vi "Teleop.vi"(10 "Match Info":T1={"Autonomous Elapsed Seconds"=0.0, "TeleOp Elapsed Seconds"=0.0, "Disabled Elapsed Seconds"=0.0, "Visited Autonomous"=FALSE, "Visited TeleOp"=FALSE, "Visited Disabled"=FALSE, "Autonomous Settings"={"Autonomous Style"=enum."Independent", "VI Refnum"=refnum}}, 11 "Call Context":T2) -> ()   [LabVIEW 2013]
doc: "This VI is called for each TeleOp packet received from the DS where the robot is not disabled. It is often used to read from the joysticks and update I/O or to update setpoints for timed control loops. It should complete and return within 20 milliseconds or it may miss DS packets."
uses:
  <vilib>/Rock Robotics/WPI/DriverStation/WPI_DriverStationDerivedRobotMode.ctl
  <vilib>/Rock Robotics/WPI/DriverStation/WPI_DriverStationMatch Info.ctl
  RefnameEnum.ctl
  LEDSaction.ctl
  Robot Global Data.vi
  <vilib>/Rock Robotics/WPI/Joystick/WPI_JoystickGetSetRefNum.vi
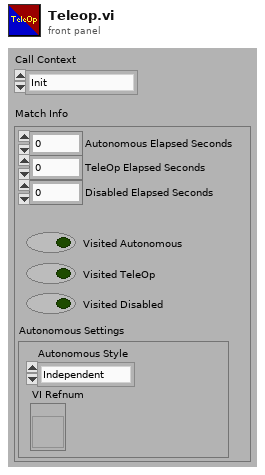
[diagram p1: front panel]
types:
  T1 = typedef "WPI_DriverStationMatch Info.ctl" = cluster{"Autonomous Elapsed Seconds":dbl, "TeleOp Elapsed Seconds":dbl, "Disabled Elapsed Seconds":dbl, "Visited Autonomous":bool, "Visited TeleOp":bool, "Visited Disabled":bool, "Autonomous Settings":cluster{"Autonomous Style":enum16{"Iterative", "Independent"}, "VI Refnum":refnum<vi>}}
  T2 = typedef "WPI_DriverStationDerivedRobotMode.ctl" = enum16{"Init", "Execute", "Stop"}
  T3 = typedef "RefnameEnum.ctl" = enum16{"TankDrive", "Controller1", "Controller2", "SonicShifter", "Compressor"}
  T4 = typedef "WPI_JoystickDevRef.ctl" = cluster{"Device":T5}
  T5 = typedef "WPI_JoystickDeviceEnum.ctl" = enum16{"USB 1", "USB 2", "USB 3", "USB 4", "Kinect 1", "Kinect 2"}
  T6 = typedef "WPI_JoystickButtonState.ctl" = cluster{"Button 1":bool, "Button 2":bool, "Button 3":bool, "Button 4":bool, "Button 5":bool, "Button 6":bool, "Button 7":bool, "Button 8":bool, "Button 9":bool, "Button 10":bool, "Button 11":bool, "Button 12":bool}
  T7 = cluster{"axis 1 (x)":dbl, "axis 2 (y)":dbl, "axis 3 (throttle)":dbl, "axis 4":dbl, "axis 5":dbl, "axis 6":dbl}
  T8 = typedef "LEDSaction.ctl" = enum16{"Init", "10SecondsLeft", "LimitDown", "LimitUp", "CollectDown", "CollectUp", "NotHot", "Hot", "Shift", "RollBack", "RollFwd", "Shoot", "Distance Low", "DistanceHigh", "PressureLow", "PressureHigh"}
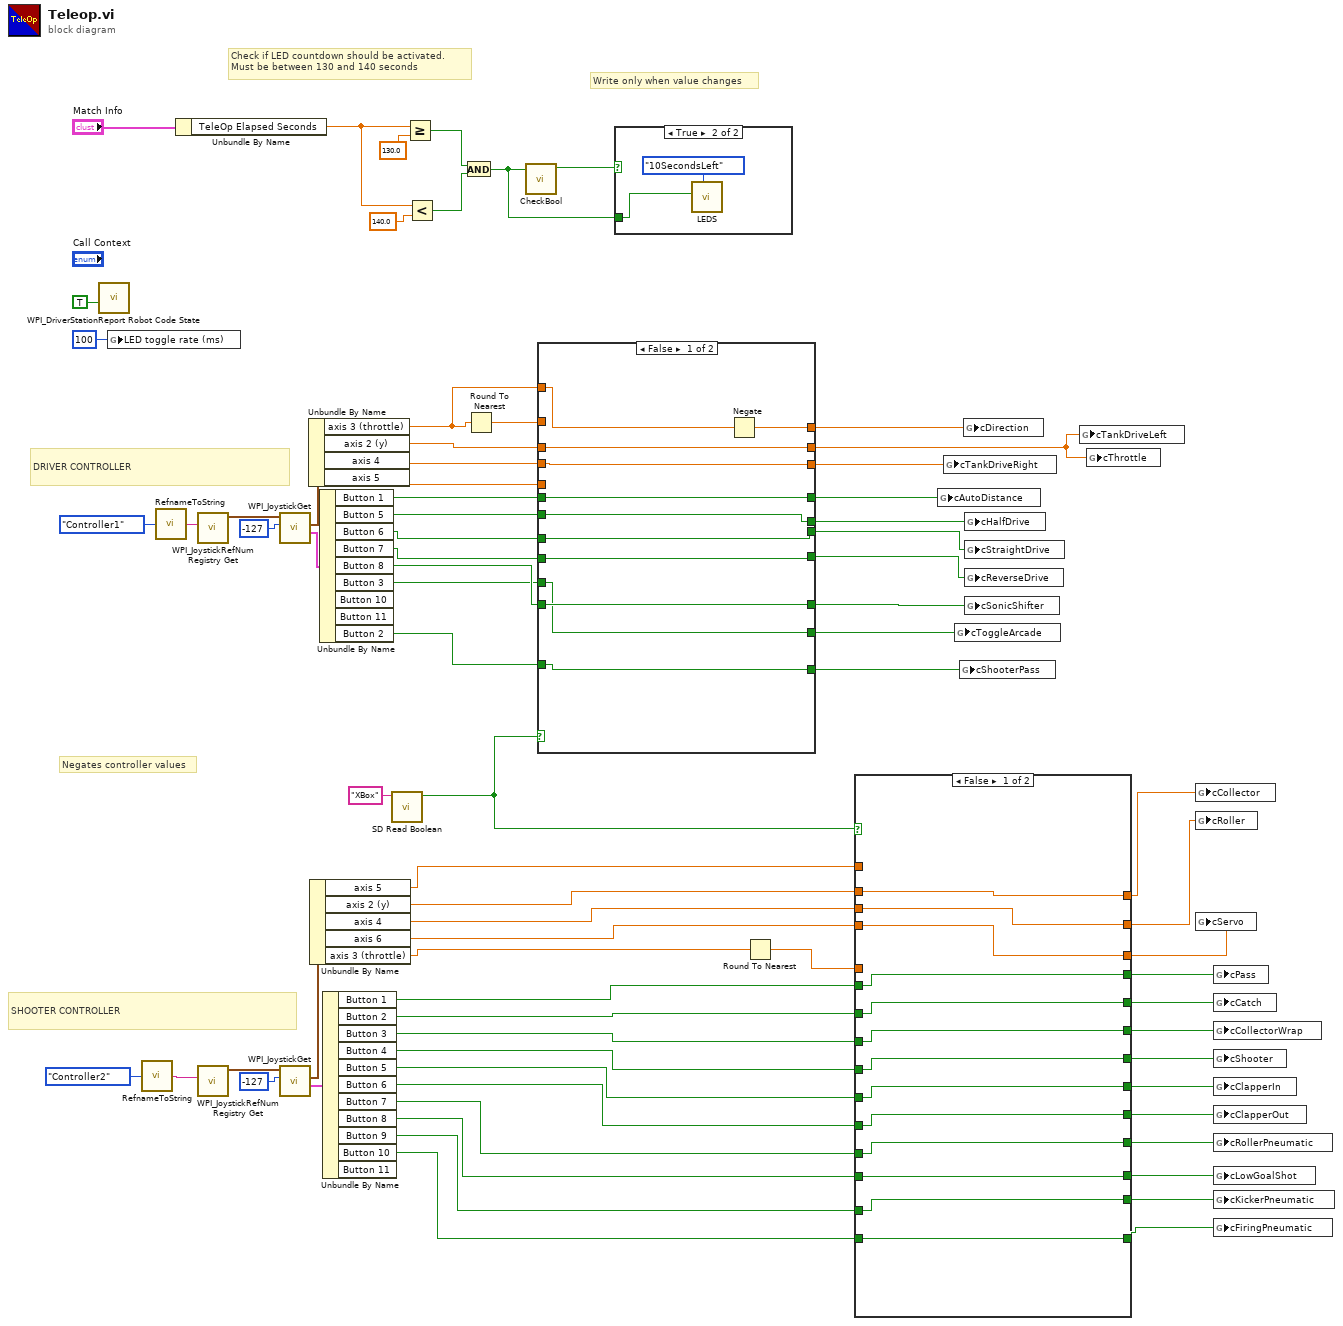
[diagram p0: block diagram]
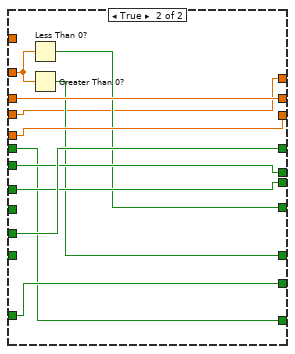
[diagram p3: hidden frame]
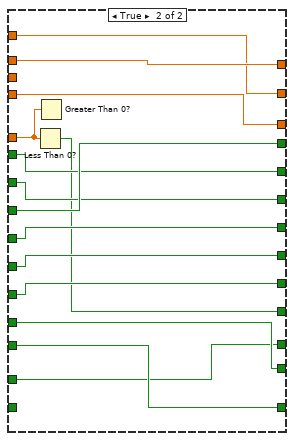
[diagram p4: hidden frame]
diagram:
  # "Write only when value changes"
  # "Check if LED countdown should be activated.\nMust be between 130 and 140 seconds"
  # "SHOOTER CONTROLLER"
  # "DRIVER CONTROLLER"
  # "Negates controller values"
  n1 = call <vilib>:"WPI_DriverStationReport Robot Code State.vi"("TeleOp"=TRUE ("Autonomous")) -> ()  [unwired: 10 in, 1 out]
  n2 = global write "Robot Global Data.vi" "LED toggle rate (ms)"(u32 100 ("LED ms toggle rate")) -> ()
  n3 = call "RefnameToString.vi"("Enum"=RefnameEnum."Controller2") -> ("Refname"=w66:string)
  n4 = call "RefnameToString.vi"("Enum"=RefnameEnum."Controller1") -> ("Refname"=w71:string)
  n5 = Unbundle By Name("Match Info") -> ("TeleOp Elapsed Seconds"=w7:dbl)
  n6 = call <vilib>:"WPI_JoystickRefNum Registry Get.vi"("refnum name"=w71) -> ("JoystickDevRef"=w73:T4)  [unwired: 1 in, 9 out]
  n7 = call <vilib>:"WPI_JoystickRefNum Registry Get.vi"("refnum name"=w66) -> ("JoystickDevRef"=w64:T4)  [unwired: 1 in, 9 out]
  n8 = call <vilib>:"WPI_JoystickGet.vi"("Scaler"=i8 -127, "JoystickDevRef"=w73) -> ("Buttons"=w68:T6, "Axes"=w69:T7)  [unwired: 4 out]
  n9 = call <vilib>:"WPI_JoystickGet.vi"("Scaler"=i8 -127, "JoystickDevRef"=w64) -> ("Buttons"=w62:T6, "Axes"=w63:T7)  [unwired: 4 out]
  n10 = Unbundle By Name(w69) -> ("axis 3 (throttle)"=w18:dbl, "axis 2 (y)"=w33:dbl, "axis 4"=w32:dbl, "axis 5"=w21:dbl)
  n11 = Unbundle By Name(w63) -> ("axis 5"=w34:dbl, "axis 2 (y)"=w42:dbl, "axis 4"=w41:dbl, "axis 6"=w40:dbl, "axis 3 (throttle)"=w39:dbl)
  n12 = Unbundle By Name(w68) -> ("Button 1"=w31:bool, "Button 5"=w28:bool, "Button 6"=w27:bool, "Button 7"=w25:bool, "Button 8"=w22:bool, "Button 3"=w20:bool, "Button 2"=w16:bool)  [unwired: 2 out]
  n13 = Unbundle By Name(w62) -> ("Button 1"=w58:bool, "Button 2"=w59:bool, "Button 3"=w60:bool, "Button 4"=w61:bool, "Button 5"=w57:bool, "Button 6"=w56:bool, "Button 7"=w55:bool, "Button 8"=w43:bool, "Button 9"=w54:bool, "Button 10"=w53:bool)  [unwired: 1 out]
  n14 = call <vilib>:"SD Read Boolean.vi"("Name"="XBox") -> ("Boolean"=w14:bool)  [unwired: 8 in, 2 out]
  n15 = Greater Or Equal?(x=w7, y=130.0) -> (x >= y?=w5:bool)
  n16 = Less?(x=w7, y=140.0) -> (x < y?=w4:bool)
  n17 = And(x=w5, y=w4) -> (x .and. y?=w2:bool)
  n18 = Round To Nearest(number=w18) -> (nearest integer value=w19:dbl)
  n19 = call "CheckBool.vi"("Input Boolean"=w2) -> ("Boolean Changed?"=w3:bool)  [unwired: 10 in]
  n20 = case shown="False" w14 {
    tunnel: w33 -> [w86 w96]
    tunnel: [w86 w96] -> w12
    tunnel: w32 -> [w85 w89]
    tunnel: [w85 w97] -> w11
    tunnel: [w84 w95] -> w30
    tunnel: w31 -> [w84 w87]
    tunnel: [w83 w94] -> w29
    tunnel: w28 -> [w83 w94]
    tunnel: [w82 w93] -> w26
    tunnel: w27 -> [w82 w93]
    tunnel: w25 -> [w81 _]
    tunnel: [w81 w91] -> w24
    tunnel: [w80 w92] -> w23
    tunnel: w22 -> [w80 _]
    tunnel: w21 -> [_ w97]
    tunnel: w20 -> [w78 w95]
    tunnel: w19 -> [_ w90]
    tunnel: [w77 w89] -> w13
    tunnel: w18 -> [w79 _]
    tunnel: [w78 w88] -> w17
    tunnel: w16 -> [w76 w88]
    tunnel: [w76 w87] -> w1
    frame False {
      n21 = Negate(x=w79) -> (-x=w77:dbl)
    }
    frame True {
      n22 = Less Than 0?(x=w90) -> (x < 0?=w91:bool)
      n23 = Greater Than 0?(x=w90) -> (x > 0?=w92:bool)
    }
  }
  n24 = case shown="True" w3 {
    tunnel: w2 -> [_ w98]
    frame False {
    }
    frame True {
      n25 = call "LEDS.vi"("Action"=LEDSaction."10SecondsLeft", "On/Off"=w98) -> ()  [unwired: 9 in, 1 out]
    }
  }
  n26 = Round To Nearest(number=w39) -> (nearest integer value=w38:dbl)
  n27 = case shown="False" w14 {
    tunnel: w61 -> [w107 w123]
    tunnel: w60 -> [w106 w126]
    tunnel: w59 -> [w105 w124]
    tunnel: w58 -> [w104 w125]
    tunnel: w57 -> [w108 w122]
    tunnel: w56 -> [w109 w121]
    tunnel: w55 -> [w110 w120]
    tunnel: w54 -> [w111 w113]
    tunnel: w53 -> [w112 _]
    tunnel: [w112 w119] -> w52
    tunnel: [w111 w120] -> w51
    tunnel: [w110 w115] -> w50
    tunnel: [w109 w121] -> w49
    tunnel: [w108 w122] -> w48
    tunnel: [w107 w123] -> w47
    tunnel: [w106 w124] -> w46
    tunnel: [w105 w125] -> w45
    tunnel: [w104 w126] -> w44
    tunnel: w43 -> [w100 w119]
    tunnel: [w103 w118] -> w37
    tunnel: w42 -> [w103 w118]
    tunnel: w41 -> [w102 _]
    tunnel: [w102 w116] -> w36
    tunnel: w40 -> [w101 w117]
    tunnel: [w101 w117] -> w35
    tunnel: w38 -> [_ w114]
    tunnel: w34 -> [_ w116]
    tunnel: [w100 w113] -> w10
    frame False {
    }
    frame True {
      n28 = Less Than 0?(x=w114) -> (x < 0?=w115:bool)
      n29 = Greater Than 0?(x=w114) -> ()  [unwired: 1 out]
    }
  }
  n30 = global write "Robot Global Data.vi" "cAutoDistance"(w30) -> ()
  n31 = global write "Robot Global Data.vi" "cTankDriveRight"(w11) -> ()
  n32 = global write "Robot Global Data.vi" "cToggleArcade"(w17) -> ()
  n33 = global write "Robot Global Data.vi" "cShooterPass"(w1) -> ()
  n34 = global write "Robot Global Data.vi" "cDirection"(w13) -> ()
  n35 = global write "Robot Global Data.vi" "cHalfDrive"(w29) -> ()
  n36 = global write "Robot Global Data.vi" "cStraightDrive"(w26) -> ()
  n37 = global write "Robot Global Data.vi" "cReverseDrive"(w24) -> ()
  n38 = global write "Robot Global Data.vi" "cSonicShifter"(w23) -> ()
  n39 = global write "Robot Global Data.vi" "cTankDriveLeft"(w12) -> ()
  n40 = global write "Robot Global Data.vi" "cThrottle"(w12) -> ()
  n41 = global write "Robot Global Data.vi" "cCollector"(w37) -> ()
  n42 = global write "Robot Global Data.vi" "cRoller"(w36) -> ()
  n43 = global write "Robot Global Data.vi" "cServo"(w35) -> ()
  n44 = global write "Robot Global Data.vi" "cPass"(w44) -> ()
  n45 = global write "Robot Global Data.vi" "cCatch"(w45) -> ()
  n46 = global write "Robot Global Data.vi" "cCollectorWrap"(w46) -> ()
  n47 = global write "Robot Global Data.vi" "cShooter"(w47) -> ()
  n48 = global write "Robot Global Data.vi" "cClapperIn"(w48) -> ()
  n49 = global write "Robot Global Data.vi" "cClapperOut"(w49) -> ()
  n50 = global write "Robot Global Data.vi" "cRollerPneumatic"(w50) -> ()
  n51 = global write "Robot Global Data.vi" "cLowGoalShot"(w10) -> ()
  n52 = global write "Robot Global Data.vi" "cKickerPneumatic"(w51) -> ()
  n53 = global write "Robot Global Data.vi" "cFiringPneumatic"(w52) -> ()
